vi "initializeKickValueTest.vi"(7 "samples":dbl, 8 "error in (no error)":errorcluster, 9 "ForceValue":T2={"delta_kick"=0.0, "kick_min"=1.0, "kick_max"=0.0}, 10 "BallValue":T1={"delta_ball"=0.0, "v_min_ball"=1.0, "v_max_ball"=0.0}, 11 "Game in":refnum<class "Game.lvclass">) -> (0 "error out":errorcluster, 2 "kickForceList":dbl[][](array[numeric]), 3 "Game out":refnum<class "Game.lvclass">)   [LabVIEW 2023, in "Game.lvclass"]
uses:
  Game.lvclass
  KickValue.ctl
  BallValue.ctl
  <vilib>/Analysis/1siggen.llb/Ramp Pattern by Delta.vi
  <vilib>/Analysis/NI_AALBase.lvlib
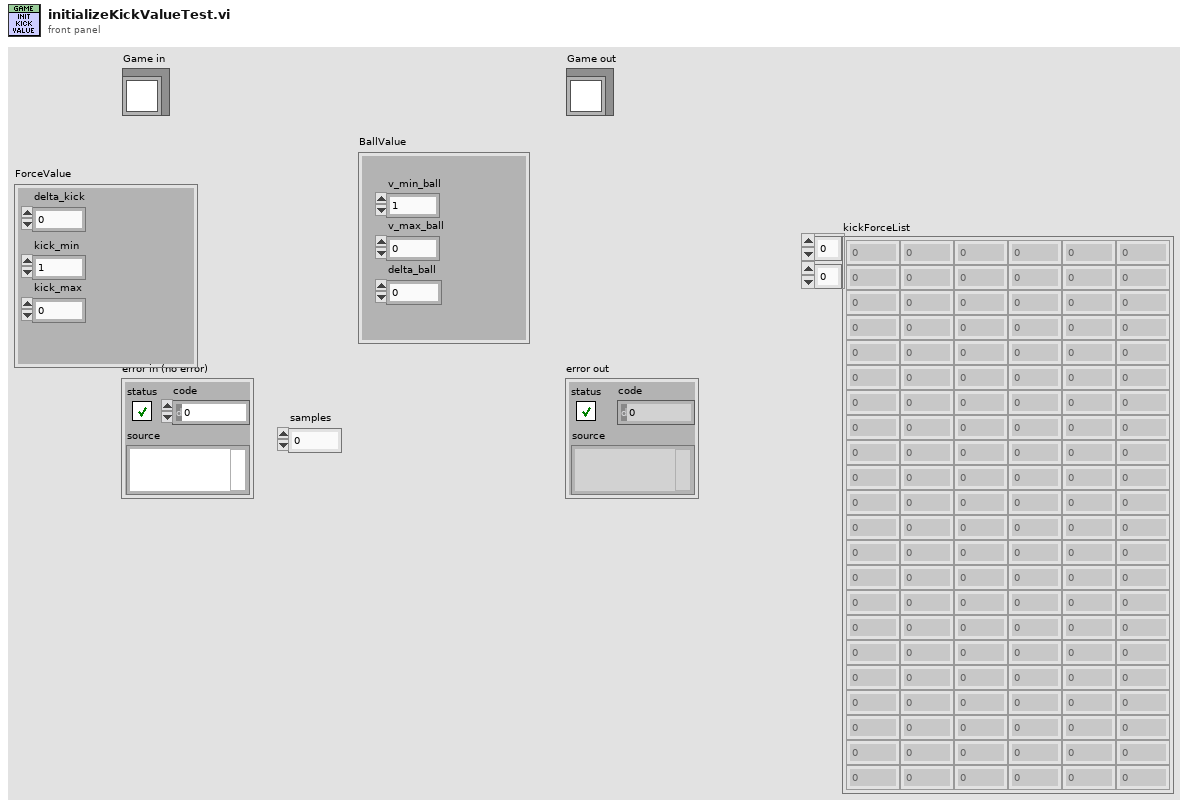
[diagram p1: front panel]
types:
  T1 = typedef "Game.lvclass/BallValue.ctl" = cluster{"delta_ball":dbl, "v_min_ball":dbl, "v_max_ball":dbl}
  T2 = typedef "Game.lvclass/KickValue.ctl" = cluster{"delta_kick":dbl, "kick_min":dbl, "kick_max":dbl}
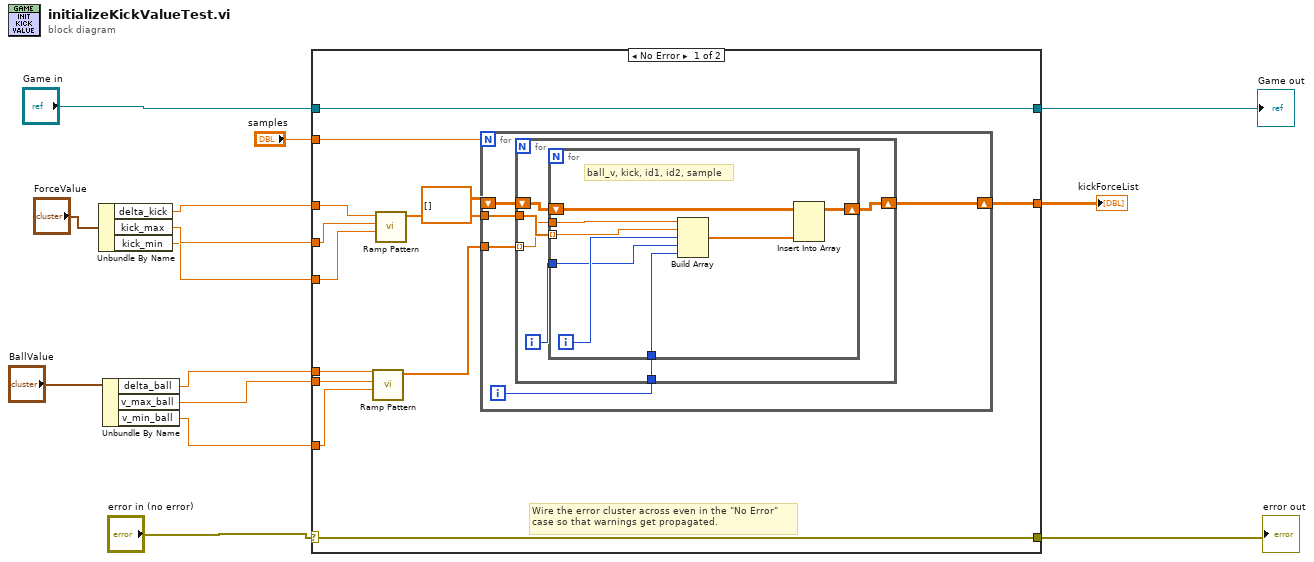
[diagram p0: block diagram]
diagram:
  n1 = Unbundle By Name("ForceValue") -> ("delta_kick"=w7:dbl, "kick_max"=w6:dbl, "kick_min"=w5:dbl)
  n2 = Unbundle By Name("BallValue") -> ("delta_ball"=w3:dbl, "v_max_ball"=w2:dbl, "v_min_ball"=w1:dbl)
  n3 = case shown="No Error" "error in (no error)" {
    selector: "error in (no error)" -> [w26 w48]
    tunnel: [w26 w48] -> w9
    tunnel: [w27 w47] -> w11
    tunnel: "Game in" -> [w27 w47]
    tunnel: w7 -> [w25 _]
    tunnel: w6 -> [w24 _]
    tunnel: w5 -> [w23 _]
    tunnel: "samples" -> [w21 _]
    tunnel: [w19 _] -> w13
    tunnel: w3 -> [w18 _]
    tunnel: w2 -> [w17 _]
    tunnel: w1 -> [w16 _]
    frame No Error {
      # "Wire the error cluster across even in the \"No Error\"\ncase so that warnings get propagated."
      n4 = call-poly <vilib>:"Ramp Pattern.vi"("start"=w16, "end"=w17, "delta"=w18) -> ("Ramp Pattern"=w15:dbl[])  [unwired: 6 in, 2 out]
      n5 = call-poly <vilib>:"Ramp Pattern.vi"("start"=w23, "end"=w24, "delta"=w25) -> ("Ramp Pattern"=w22:dbl[])  [unwired: 6 in, 2 out]
      n6 = for {
        N: w21 -> [_]
        tunnel: w22 -> [w32]
        shift-right: [w30] -> w19
        shift-left: dbl[][] [] -> [w29]
        tunnel: w15 -> [w28]
        i -> [w31]
        n7 = for {
          tunnel: w32 -> [w38]
          tunnel: w31 -> [w33]
          tunnel: w28 -> [w35] mode=indexing
          shift-right: [w37] -> w30
          shift-left: w29 -> [w36]
          i -> [w34]
          n8 = for {
            tunnel: w38 -> [w46] mode=indexing
            shift-right: [w43] -> w37
            shift-left: w36 -> [w42]
            tunnel: w35 -> [w41]
            tunnel: w34 -> [w40]
            tunnel: w33 -> [w39]
            i -> [w45]
            # "ball_v, kick, id1, id2, sample"
            n9 = Build Array(w41, w46, w45, w40, w39) -> (w44:dbl[])
            n10 = Insert Into Array(array=w42, new element=w44) -> (w43:dbl[][])  [unwired: 2 in]
          }
        }
      }
    }
    frame Error {
    }
  }
  "error out" <- w9
  "Game out" <- w11
  "kickForceList" <- w13
